vi "PathPlanner_ObstacleGrid_FromJSON.vi"(11 "JSON String":string) -> (0 "Error":bool, 3 "PathPlanner_Grid":T1)   [LabVIEW 2019, in "PathPlanner24.lvlib"]
doc: "Parse an obstacle grid from a JSON formatted string. \n\nInputs: \n - JSON String - string- The string containing the obstacle grid definition.\n\nOutputs:\n - PathPlanner_ObstacleGrid - cluster - Obstacle grid read from JSON file.\n - Error - boolean - TRUE if an error occured."
uses:
  PathPlanner24.lvlib
  TypeDef/PathPlannerObstacleGrid.ctl
panel:
  in  "field_size":cluster{"x":dbl, "y":dbl}
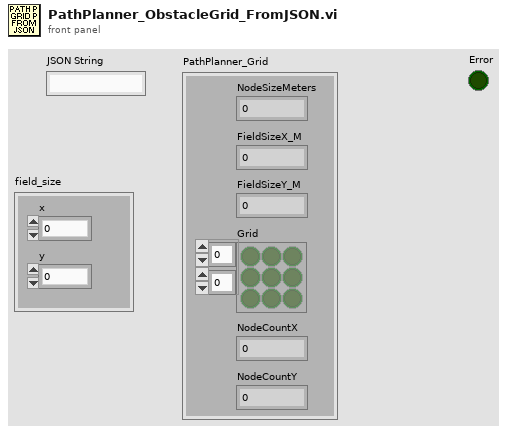
[diagram p1: front panel]
types:
  T1 = typedef "PathPlanner24.lvlib/PathPlannerObstacleGrid.ctl" = cluster{"NodeSizeMeters":dbl, "Grid":bool[][], "NodeCountX":i32, "NodeCountY":i32, "FieldSizeX_M":dbl, "FieldSizeY_M":dbl}
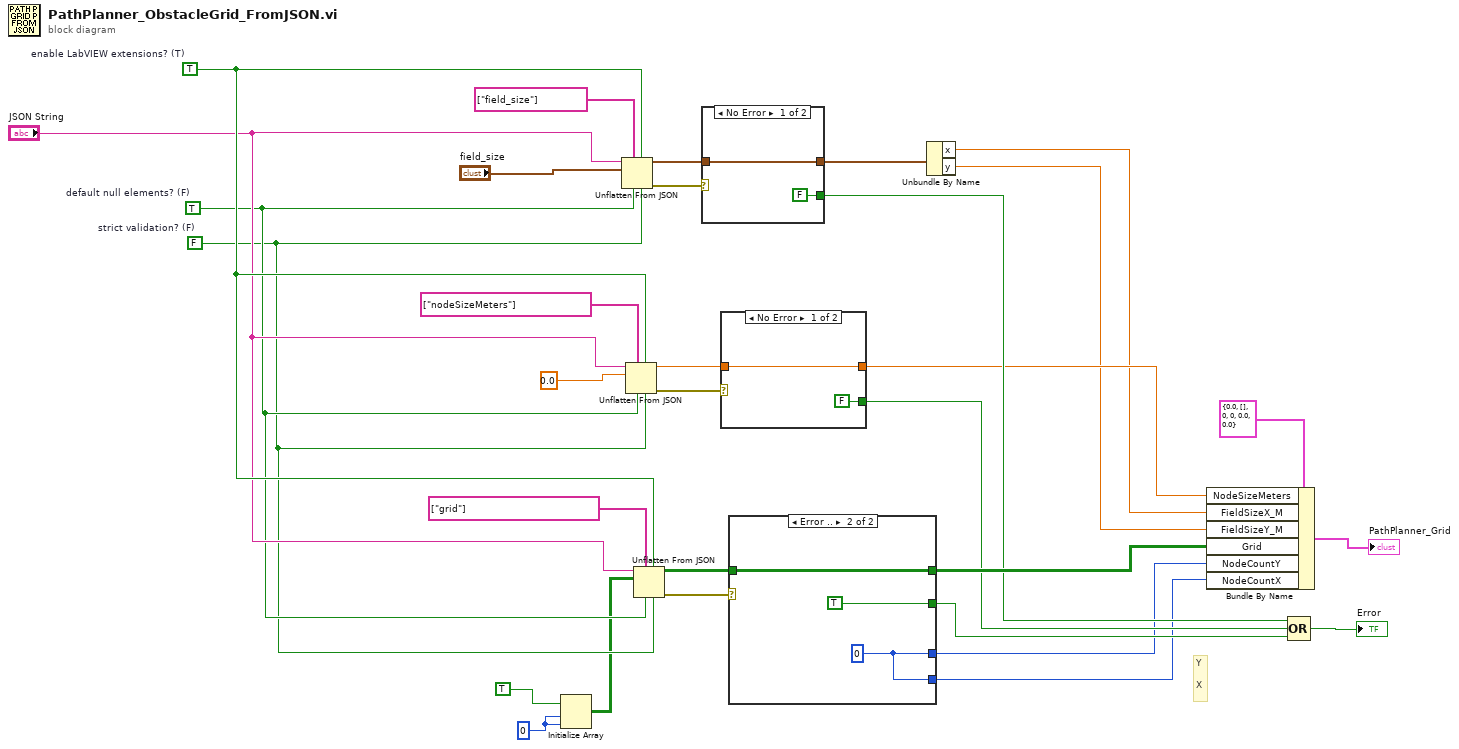
[diagram p0: block diagram]
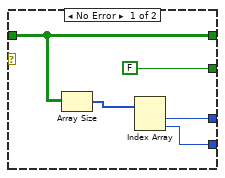
[diagram p2: hidden frame]
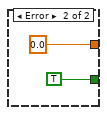
[diagram p3: hidden frame]
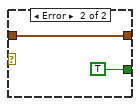
[diagram p4: hidden frame]
diagram:
  w16 = 0 ("dimension size")
  w17 = FALSE  # strict validation? (F)
  w18 = TRUE  # default null elements? (F)
  w20 = TRUE  # enable LabVIEW extensions? (T)
  # "Y \n\nX"
  n1 = Initialize Array(TRUE, w16, w16) -> (w15:bool[][])
  n2 = Unflatten From JSON(path=string[] ["field_size"] ("path 3"), enable LabVIEW extensions? (T)=w20, JSON string="JSON String", type and defaults="field_size", default null elements? (F)=w18, strict validation? (F)=w17) -> (value=w28:cluster{"x":dbl, "y":dbl}, error out=w29:errorcluster)  [unwired: 1 in]
  n3 = Unflatten From JSON(path=string[] ["nodeSizeMeters"] ("path 3"), enable LabVIEW extensions? (T)=w20, JSON string="JSON String", type and defaults=0.0, default null elements? (F)=w18, strict validation? (F)=w17) -> (value=w26:dbl, error out=w27:errorcluster)  [unwired: 1 in]
  n4 = Unflatten From JSON(path=string[] ["grid"] ("path 3"), enable LabVIEW extensions? (T)=w20, JSON string="JSON String", type and defaults=w15, default null elements? (F)=w18, strict validation? (F)=w17) -> (value=w21:bool[][], error out=w22:errorcluster)  [unwired: 1 in]
  n5 = case shown="No Error" w29 {
    tunnel: w28 -> [w33 w35]
    tunnel: [w33 w35] -> w11
    tunnel: [FALSE TRUE] -> w8
    frame No Error {
    }
    frame Error {
    }
  }
  n6 = case shown="No Error" w27 {
    tunnel: w26 -> [w37 _]
    tunnel: [w37 0.0] -> w3
    tunnel: [FALSE TRUE] -> w7
    frame No Error {
    }
    frame Error {
    }
  }
  n7 = case shown="Error .." w22 {
    tunnel: w21 -> [w43 w47]
    tunnel: [w43 w47] -> w10
    tunnel: [FALSE TRUE] -> w9
    tunnel: [w41 w45] -> w5
    tunnel: [w40 w45] -> w4
    frame No Error {
      n8 = Array Size(array=w43) -> (size(s)=w42:i32[])
      n9 = Index Array(array=w42) -> (element #1=w41:i32, element #2=w40:i32)  [unwired: 2 in]
    }
    frame Error {
      w45 = 0
    }
  }
  n10 = Unbundle By Name(w11) -> ("x"=w2:dbl, "y"=w1:dbl)
  n11 = Bundle By Name(cluster=T1 {"NodeSizeMeters"=0.0, "Grid"=[], "NodeCountX"=0, "NodeCountY"=0, "FieldSizeX_M"=0.0, "FieldSizeY_M"=0.0} ("PathPlanner_Grid"), "NodeSizeMeters"=w3, "FieldSizeX_M"=w2, "FieldSizeY_M"=w1, "Grid"=w10, "NodeCountY"=w5, "NodeCountX"=w4) -> (→"PathPlanner_Grid":T1)
  n12 = Compound Arithmetic op=OR(w8, w7, w9) -> (→"Error":bool)
